vi "Calibration Convert String to String.vi"(8 "error in (no error)":errorcluster, 10 "all rows":string[](array[string]), 11 "Serial Number in":T1) -> (0 "error out":errorcluster, 2 "size(s)":i32, 3 "Serial Number out":T1)   [LabVIEW 2016]
uses:
  Type Definitions/Calibration SN.ctl
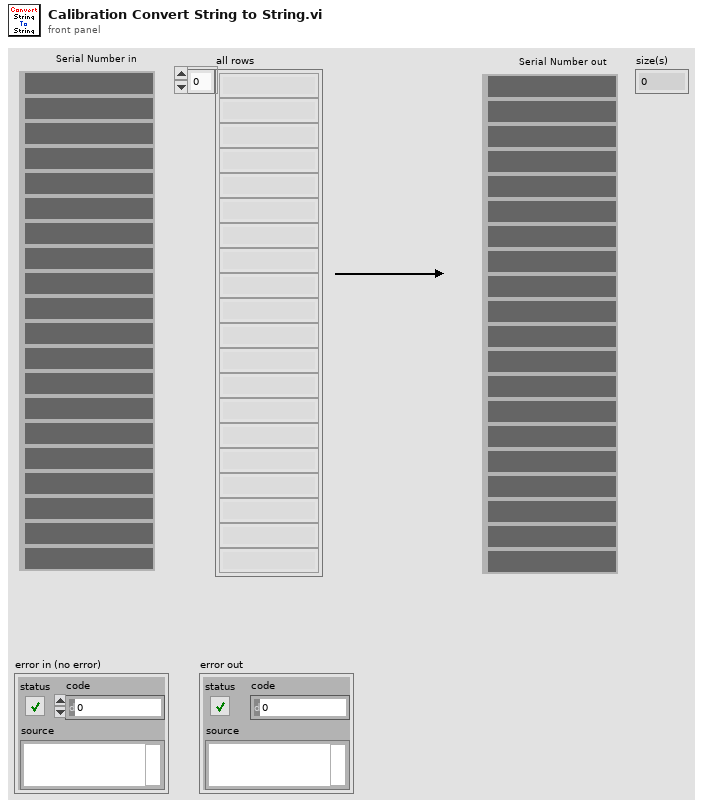
[diagram p1: front panel]
types:
  T1 = typedef "Calibration SN.ctl" = cluster{"Eq 1":string, "Eq 2":string, "Eq 3":string, "Eq 4":string, "Eq 5":string, "Eq 6":string, "Eq 7":string, "Eq 8":string, "Eq 9":string, "Eq 10":string, "Eq 11":string, "Eq 12":string, "Eq 13":string, "Eq 14":string, "Eq 15":string, "Eq 16":string, "Eq 17":string, "Eq 18":string, "Eq 19":string, "Eq 20":string}
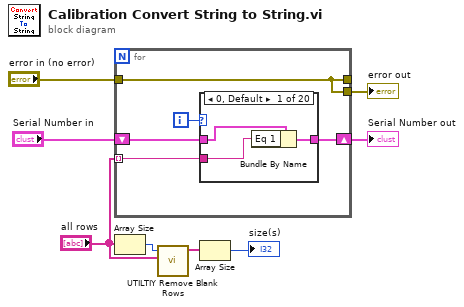
[diagram p0: block diagram]
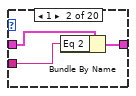
[diagram p2: hidden frame]
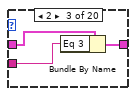
[diagram p3: hidden frame]
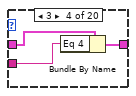
[diagram p4: hidden frame]
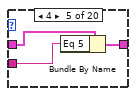
[diagram p5: hidden frame]
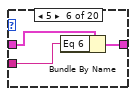
[diagram p6: hidden frame]
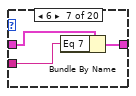
[diagram p7: hidden frame]
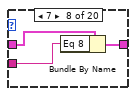
[diagram p8: hidden frame]
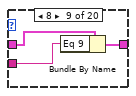
[diagram p9: hidden frame]
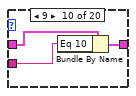
[diagram p10: hidden frame]
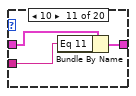
[diagram p11: hidden frame]
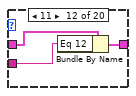
[diagram p12: hidden frame]
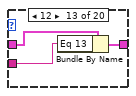
[diagram p13: hidden frame]
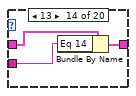
[diagram p14: hidden frame]
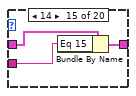
[diagram p15: hidden frame]
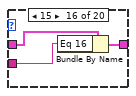
[diagram p16: hidden frame]
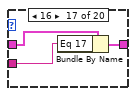
[diagram p17: hidden frame]
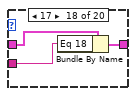
[diagram p18: hidden frame]
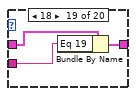
[diagram p19: hidden frame]
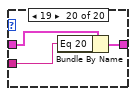
[diagram p20: hidden frame]
diagram:
  n1 = for {
    tunnel: "all rows" -> [w10] mode=indexing
    shift-right: [w11] -> w7
    shift-left: "Serial Number in" -> [w12]
    tunnel: [w9] -> _
    tunnel: "error in (no error)" -> [w9]
    tunnel: [w9] -> w5
    i -> [w13]
    n2 = case shown="0, Default" w13 {
      tunnel: w12 -> [w16 w19 w22 w25 w28 w31 w34 w37 w40 w43 w46 w49 w52 w55 w58 w61 w63 w66 w69 w72]
      tunnel: [w15 w18 w21 w24 w27 w30 w33 w36 w39 w42 w45 w48 w51 w54 w57 w59 w62 w65 w68 w71] -> w11
      tunnel: w10 -> [w14 w17 w20 w23 w26 w29 w32 w35 w38 w41 w44 w47 w50 w53 w56 w60 w64 w67 w70 w73]
      frame 0, Default {
        n3 = Bundle By Name(cluster=w16, "Eq 1"=w14) -> (w15:T1)
      }
      frame 1 {
        n4 = Bundle By Name(cluster=w19, "Eq 2"=w17) -> (w18:T1)
      }
      frame 2 {
        n5 = Bundle By Name(cluster=w22, "Eq 3"=w20) -> (w21:T1)
      }
      frame 3 {
        n6 = Bundle By Name(cluster=w25, "Eq 4"=w23) -> (w24:T1)
      }
      frame 4 {
        n7 = Bundle By Name(cluster=w28, "Eq 5"=w26) -> (w27:T1)
      }
      frame 5 {
        n8 = Bundle By Name(cluster=w31, "Eq 6"=w29) -> (w30:T1)
      }
      frame 6 {
        n9 = Bundle By Name(cluster=w34, "Eq 7"=w32) -> (w33:T1)
      }
      frame 7 {
        n10 = Bundle By Name(cluster=w37, "Eq 8"=w35) -> (w36:T1)
      }
      frame 8 {
        n11 = Bundle By Name(cluster=w40, "Eq 9"=w38) -> (w39:T1)
      }
      frame 9 {
        n12 = Bundle By Name(cluster=w43, "Eq 10"=w41) -> (w42:T1)
      }
      frame 10 {
        n13 = Bundle By Name(cluster=w46, "Eq 11"=w44) -> (w45:T1)
      }
      frame 11 {
        n14 = Bundle By Name(cluster=w49, "Eq 12"=w47) -> (w48:T1)
      }
      frame 12 {
        n15 = Bundle By Name(cluster=w52, "Eq 13"=w50) -> (w51:T1)
      }
      frame 13 {
        n16 = Bundle By Name(cluster=w55, "Eq 14"=w53) -> (w54:T1)
      }
      frame 14 {
        n17 = Bundle By Name(cluster=w58, "Eq 15"=w56) -> (w57:T1)
      }
      frame 15 {
        n18 = Bundle By Name(cluster=w61, "Eq 16"=w60) -> (w59:T1)
      }
      frame 16 {
        n19 = Bundle By Name(cluster=w63, "Eq 17"=w64) -> (w62:T1)
      }
      frame 17 {
        n20 = Bundle By Name(cluster=w66, "Eq 18"=w67) -> (w65:T1)
      }
      frame 18 {
        n21 = Bundle By Name(cluster=w69, "Eq 19"=w70) -> (w68:T1)
      }
      frame 19 {
        n22 = Bundle By Name(cluster=w72, "Eq 20"=w73) -> (w71:T1)
      }
    }
  }
  "Serial Number out" <- w7
  "error out" <- w5
  n23 = Array Size(array="all rows") -> (size(s)=w3:i32)
  n24 = call "UTILTIY Remove Blank Rows.vi"("all rows in"="all rows", "Numeric"=w3) -> ("all rows out"=w2:string[])  [unwired: 9 in]
  n25 = Array Size(array=w2) -> (size(s)=→"size(s)":i32)
